vi "Host Main.vi"() -> ()   [LabVIEW 2016]
panel:
  in  "?":bool
  in  "Enter Mode":bool
  in  "Select Mode of Operation":u16(ring) items=["Brute Force ", "Karplus-Strong Guitar", "Midi Utilised"]
  # "AIR MUSIC"
  # "Before running this VI ensure that \n\"Main VI\" on the myRio Target is \nalready running."
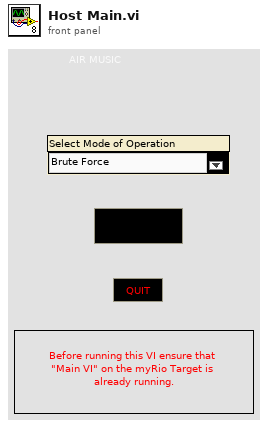
[diagram p1: front panel]
types:
  T1 = enum32{"Invalid", "Standard", "Closed", "Hidden", "Minimized", "Maximized"}
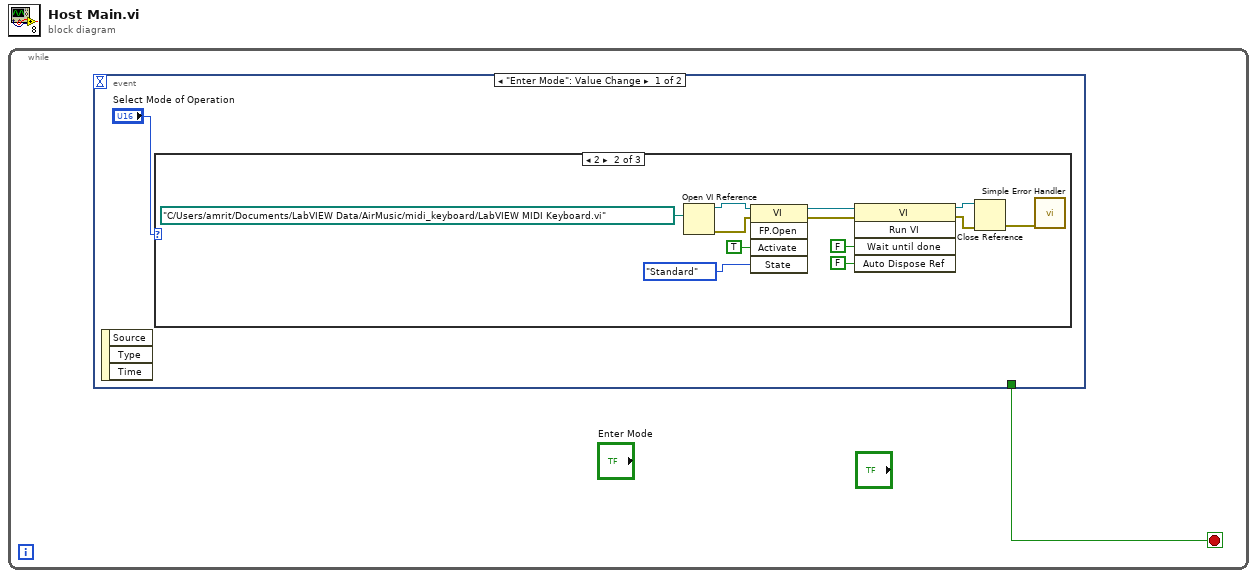
[diagram p0: block diagram]
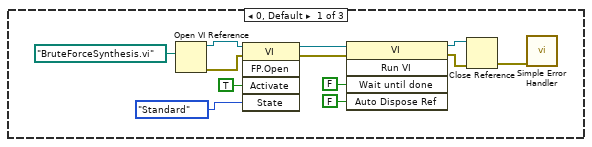
[diagram p2: hidden frame]
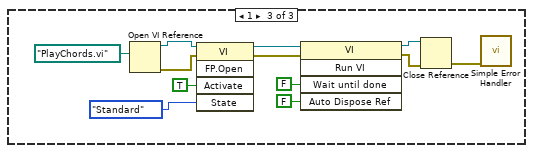
[diagram p3: hidden frame]
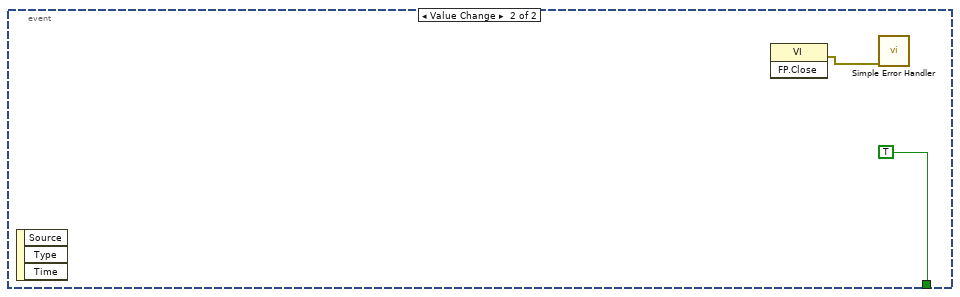
[diagram p4: hidden frame]
diagram:
  n1 = while {
    stop <- w1 stop-if-true
    n2 = event shown="[0] \"Enter Mode\": Value Change" {
      selector: _ -> [_ _]
      dyn-events: _ -> [_ _]
      timeout: _ -> [_ _]
      tunnel: [_ TRUE] -> w1
      event "Enter Mode": Value Change {
        n3 = event-data() -> ()  [unwired: 1 in, 3 out]
        n4 = case shown="2" "Select Mode of Operation" {
          frame 0, Default {
            n5 = Open VI Reference(vi path=path "BruteForceSynthesis.vi") -> (vi reference=w10:refnum<vi>, error out=w9:errorcluster)  [unwired: 5 in]
            n6 = invoke class="VI" method="FP.Open"(reference=w10, error in=w9, "Activate"=TRUE ("Activate?"), "State"=T1."Standard") -> (reference out=w13:refnum<vi>, error out=w12:errorcluster)  [unwired: 1 in, 3 out]
            n7 = invoke class="VI" method="Run VI"(reference=w13, error in=w12, "Wait until done"=FALSE ("Wait Until Done"), "Auto Dispose Ref"=FALSE ("Auto Dispose Reference")) -> (reference out=w5:refnum<vi>, error out=w4:errorcluster)  [unwired: 1 in, 3 out]
            n8 = Close Reference(reference=w5, error in (no error)=w4) -> (error out=w3:errorcluster)
            n9 = call <vilib>:"Simple Error Handler.vi"("error in (no error)"=w3) -> ()  [unwired: 4 in, 5 out]
          }
          frame 2 {
            n10 = Open VI Reference(vi path=path "C:/Users/amrit/Documents/LabVIEW Data/AirMusic/midi_keyboard/LabVIEW MIDI Keyboard.vi") -> (vi reference=w19:refnum<vi>, error out=w20:errorcluster)  [unwired: 5 in]
            n11 = invoke class="VI" method="FP.Open"(reference=w19, error in=w20, "Activate"=TRUE ("Activate?"), "State"=T1."Standard") -> (reference out=w16:refnum<vi>, error out=w17:errorcluster)  [unwired: 1 in, 3 out]
            n12 = invoke class="VI" method="Run VI"(reference=w16, error in=w17, "Wait until done"=FALSE ("Wait Until Done"), "Auto Dispose Ref"=FALSE ("Auto Dispose Reference")) -> (reference out=w24:refnum<vi>, error out=w25:errorcluster)  [unwired: 1 in, 3 out]
            n13 = Close Reference(reference=w24, error in (no error)=w25) -> (error out=w26:errorcluster)
            n14 = call <vilib>:"Simple Error Handler.vi"("error in (no error)"=w26) -> ()  [unwired: 4 in, 5 out]
          }
          frame 1 {
            n15 = Open VI Reference(vi path=path "PlayChords.vi") -> (vi reference=w31:refnum<vi>, error out=w32:errorcluster)  [unwired: 5 in]
            n16 = invoke class="VI" method="FP.Open"(reference=w31, error in=w32, "Activate"=TRUE ("Activate?"), "State"=T1."Standard") -> (reference out=w28:refnum<vi>, error out=w29:errorcluster)  [unwired: 1 in, 3 out]
            n17 = invoke class="VI" method="Run VI"(reference=w28, error in=w29, "Wait until done"=FALSE ("Wait Until Done"), "Auto Dispose Ref"=FALSE ("Auto Dispose Reference")) -> (reference out=w36:refnum<vi>, error out=w37:errorcluster)  [unwired: 1 in, 3 out]
            n18 = Close Reference(reference=w36, error in (no error)=w37) -> (error out=w38:errorcluster)
            n19 = call <vilib>:"Simple Error Handler.vi"("error in (no error)"=w38) -> ()  [unwired: 4 in, 5 out]
          }
        }
      }
      event Value Change {
        n20 = event-data() -> ()  [unwired: 1 in, 3 out]
        n21 = invoke class="VI" method="FP.Close"() -> (error out=w39:errorcluster)  [unwired: 3 in, 2 out]
        n22 = call <vilib>:"Simple Error Handler.vi"("error in (no error)"=w39) -> ()  [unwired: 4 in, 5 out]
      }
    }
  }
